vi "Time FGV.vi"(7 "Set/Get":enum16{"Set", "Get"}(ring), 8 "error in (no error)":errorcluster, 10 "Target":dbl, 11 "Elevator Controller Actor in":refnum<class "Elevator Controller Actor.lvclass">) -> (0 "error out":errorcluster, 2 "Elapsed Time":dbl, 3 "Elevator Controller Actor out":refnum<class "Elevator Controller Actor.lvclass">)   [LabVIEW 2019]
uses:
  Elevator Controller Actor.lvclass
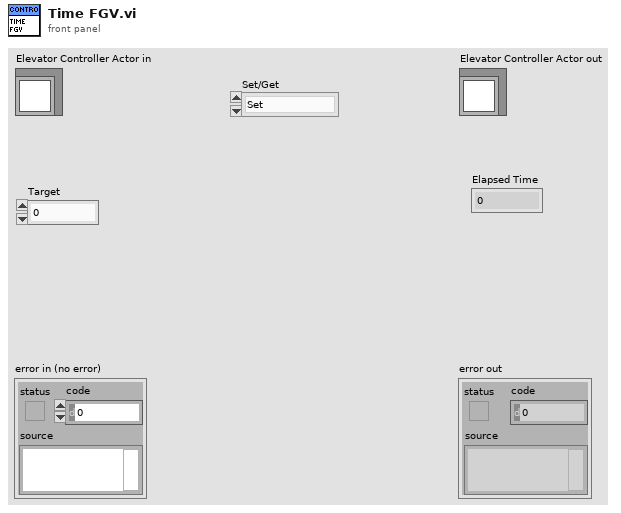
[diagram p1: front panel]
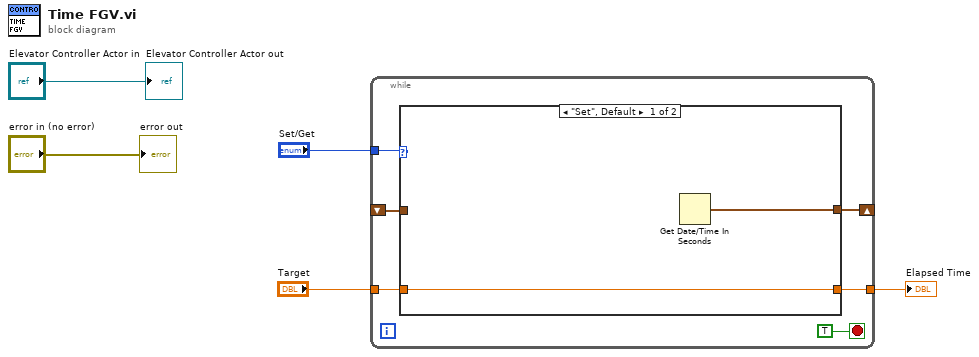
[diagram p0: block diagram]
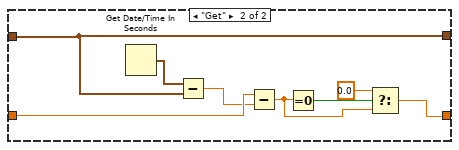
[diagram p2: hidden frame]
diagram:
  n1 = while {
    tunnel: "Set/Get" -> [w10]
    tunnel: "Target" -> [w9]
    shift-right: [w7] -> _
    shift-left: _ -> [w8]
    tunnel: [w6] -> w1
    stop <- TRUE stop-if-true
    n2 = case shown="\"Set\", Default" w10 {
      tunnel: w9 -> [w12 w19]
      tunnel: w8 -> [_ w20]
      tunnel: [w13 w20] -> w7
      tunnel: [w12 w14] -> w6
      frame "Set", Default {
        n3 = Get Date/Time In Seconds() -> (seconds since 1Jan1904=w13:timestamp)
      }
      frame "Get" {
        n4 = Get Date/Time In Seconds() -> (seconds since 1Jan1904=w21:timestamp)
        n5 = Subtract(x=w21, y=w20) -> (x-y=w18:dbl)
        n6 = Subtract(x=w19, y=w18) -> (x-y=w15:dbl)
        n7 = Equal To 0?(x=w15) -> (x = 0?=w17:bool)
        n8 = Select(t=0.0, s=w17, f=w15) -> (s? t:f=w14:dbl)
      }
    }
  }
  "Elapsed Time" <- w1
  "error out" <- "error in (no error)"
  "Elevator Controller Actor out" <- "Elevator Controller Actor in"
